vi "CohortDemo.vi"(1 "EP 1":T3={"0"=2, "1"=0, "2"=0, "3"=0, "4"=0, "5"=2, "6"=1, "7"=0, "8"=0, "9"=0, "10"=0, "11"=2, "12"=0, "13"=0, "14"=0, "15"=0}) -> ()   [LabVIEW 2012, in "Cohort.lvclass"]
uses:
  Cohort.lvclass
  PulseConfig.ctl
  StimulCtrls.lvlib
  CohortPanel.ctl
  AmplitudePanel.ctl
panel:
  out "Cohort Signal":dbl[](array[numeric])
  out "Cohort Waveform":waveform(dbl)(graph)
  in  "Sampling Frequency [Hz]":u32 format="%.2p"
  out "error out":errorcluster
  in  "Voltage Control":T1={"0"=2, "1"=2, "2"=2, "3"=2, "4"=2, "5"=2, "6"=2, "7"=2, "8"=2, "9"=2, "10"=2, "11"=2, "12"=2, "13"=2, "14"=2, "15"=2} {"15" scale=0.0..10.0; "14" scale=0.0..10.0; "13" scale=0.0..10.0; "12" scale=0.0..10.0; "11" scale=0.0..10.0; "10" scale=0.0..10.0; "9" scale=0.0..10.0; "8" scale=0.0..10.0; "7" scale=0.0..10.0; "6" scale=0.0..10.0; "5" scale=0.0..10.0; "4" scale=0.0..10.0; "3" scale=0.0..10.0; "2" scale=0.0..10.0; "1" scale=0.0..10.0; "0" scale=0.0..10.0}
  in  "Set Voltages":bool
  in  "Pulse configuration":T2={"Charge Balance"=TRUE, "Signal Amplitude"=10, "Signal Frequency [Hz]"=10, "Signal Duration [s]"=1.0, "Delay Time [s]"=0.0, "Pulse Width [s]"=0.005} {"Pulse Width [s]" format="%0.2p"; "Delay Time [s]" format="%0.2p"; "Signal Amplitude" format="%0.0p"; "Signal Duration [s]" format="%0.2p"}
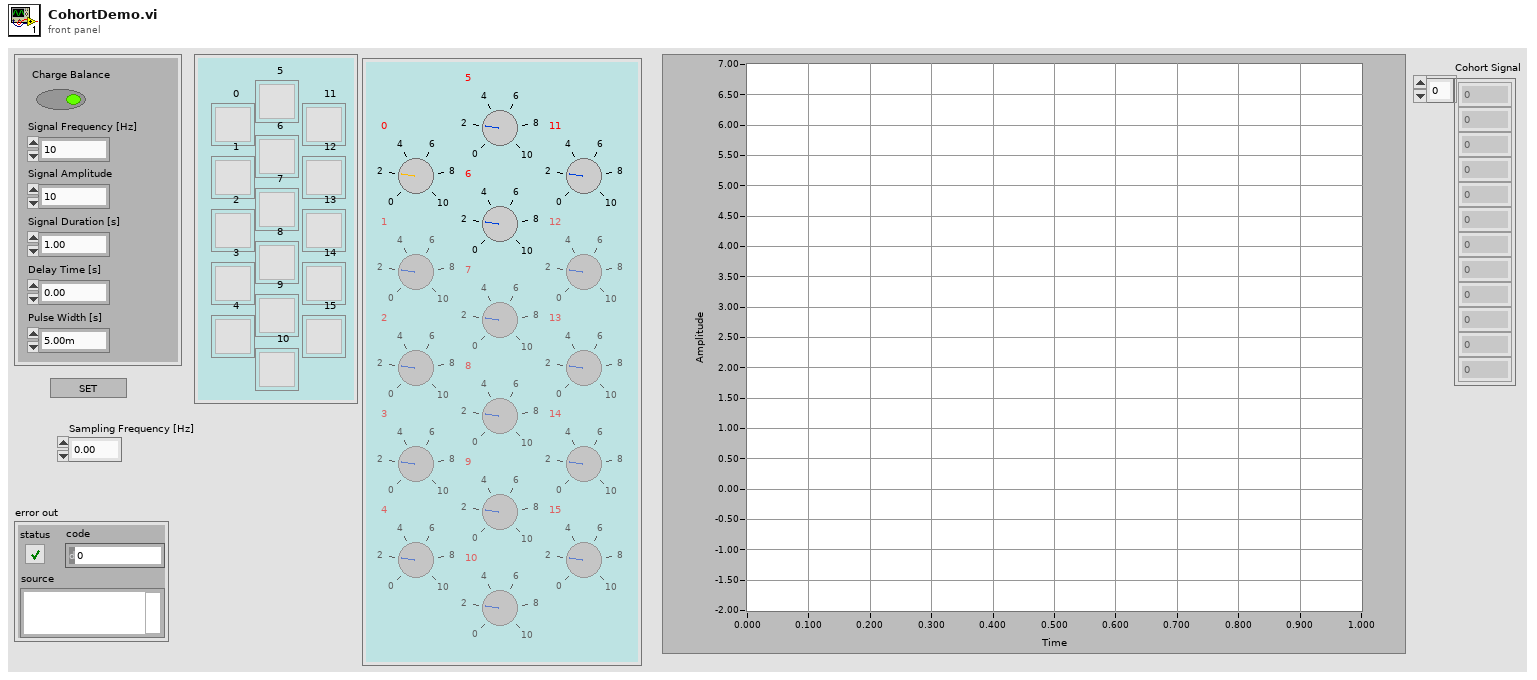
[diagram p1: front panel]
types:
  T1 = typedef "StimulCtrls.lvlib/AmplitudePanel.ctl" = cluster{"0":u16, "1":u16, "2":u16, "3":u16, "4":u16, "5":u16, "6":u16, "7":u16, "8":u16, "9":u16, "10":u16, "11":u16, "12":u16, "13":u16, "14":u16, "15":u16}
  T2 = typedef "StimulCtrls.lvlib/PulseConfig.ctl" = cluster{"Charge Balance":bool, "Signal Amplitude":u32, "Signal Frequency [Hz]":u8, "Signal Duration [s]":sgl, "Delay Time [s]":sgl, "Pulse Width [s]":sgl}
  T3 = typedef "StimulCtrls.lvlib/CohortPanel.ctl" = cluster{"0":u16, "1":u16, "2":u16, "3":u16, "4":u16, "5":u16, "6":u16, "7":u16, "8":u16, "9":u16, "10":u16, "11":u16, "12":u16, "13":u16, "14":u16, "15":u16}
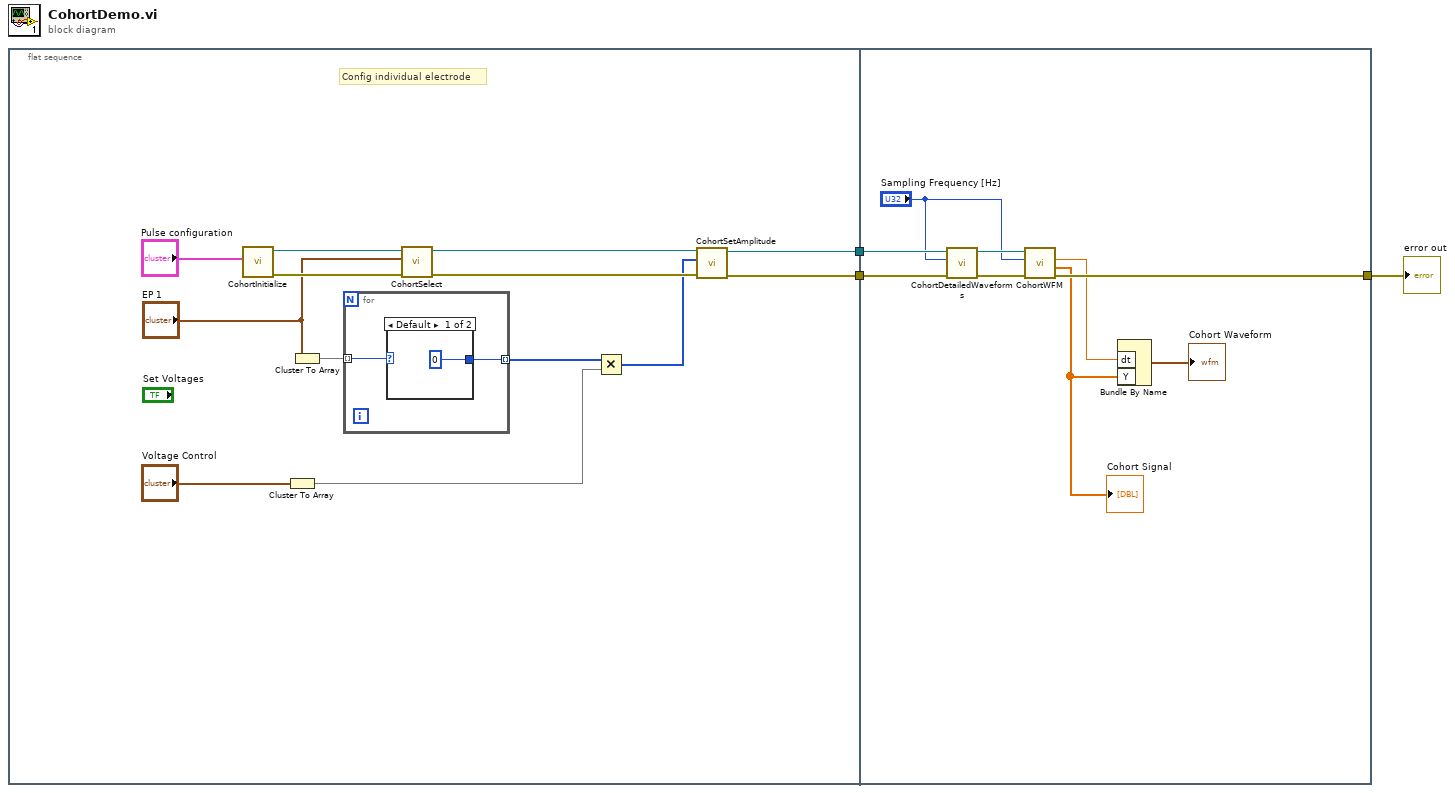
[diagram p0: block diagram]
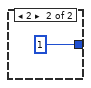
[diagram p2: hidden frame]
diagram:
  n1 = flat-sequence {
    tunnel: [w5] -> w2
    tunnel: [w4] -> w1
    tunnel: [w25] -> w3
    tunnel: w2 -> [w28]
    tunnel: w1 -> [w29]
    frame #0 {
      # "Config individual electrode"
      n2 = call "CohortInitialize.vi"("Pulse Configuration"="Pulse configuration") -> ("error out"=w15:errorcluster, "Cohort out"=w16:refnum<class "Cohort.lvclass">)  [unwired: 9 in]
      n3 = Cluster To Array(cluster="Voltage Control") -> (array=w8:u16[])
      n4 = Cluster To Array(cluster="EP 1") -> (array=w13:u16[])
      n5 = for {
        tunnel: w13 -> [w18] mode=indexing
        tunnel: [w17] -> w9 mode=indexing
        n6 = case shown="Default" w18 {
          tunnel: [0 1] -> w17
          frame Default {
          }
          frame 2 {
          }
        }
      }
      n7 = call-dynamic "CohortSelect.vi"("error in (no error)"=w15, "Electrode Panel"="EP 1", "Cohort in"=w16) -> ("error out"=w10:errorcluster, "Cohort out"=w11:refnum<class "Cohort.lvclass">)  [unwired: 7 in]
      n8 = Multiply ("Multiply.vi")(x=w9, y=w8) -> (x*y=w7:i32[])
      n9 = call-dynamic "CohortSetAmplitude.vi"("error in (no error)"=w10, "Electrode Amplitudes"=w7, "Cohort in"=w11) -> ("error out"=w5:errorcluster, "Cohort out"=w4:refnum<class "Cohort.lvclass">)  [unwired: 7 in]
    }
    frame #1 {
      n10 = call "CohortDetailedWaveforms.vi"("Cohort in"=w29, "Sampling Frequency [Hz]"="Sampling Frequency [Hz]", "error in (no error)"=w28) -> ("Cohort out"=w26:refnum<class "Cohort.lvclass">, "error out"=w27:errorcluster)  [unwired: 6 in]
      n11 = call-dynamic "CohortWFM.vi"("error in (no error)"=w27, "Sampling Frequency [Hz]"="Sampling Frequency [Hz]", "Cohort in"=w26) -> ("error out"=w25:errorcluster, "Cohort Signal"=w22:dbl[], "dt"=w21:sgl)  [unwired: 5 in, 1 out]
      "Cohort Signal" <- w22
      n12 = Bundle By Name("dt"=w21, "Y"=w22) -> (→"Cohort Waveform":waveform(dbl))  [unwired: 1 in]
    }
  }
  "error out" <- w3
